vi "power data.vi"() -> ()   [LabVIEW 2014]
uses:
  <vilib>/Rock Robotics/Network Tables/NT Read Boolean Array.vi
  <vilib>/Rock Robotics/Network Tables/NT Write Boolean Array.vi
  <vilib>/Rock Robotics/Network Tables/NT Write Numeric Array.vi
  <vilib>/Rock Robotics/WPI/Power/WPI_Power Get 6Volt Rail Voltage and Current.vi
  <vilib>/Rock Robotics/WPI/Power/WPI_Power Get 5Volt Rail Voltage and Current.vi
  <vilib>/Rock Robotics/WPI/Power/WPI_Power Get 3Volt Rail Voltage and Current.vi
  typedefs/dashboard/power data.ctl
  <vilib>/Rock Robotics/Network Tables/NT Write String.vi
panel:
  out "OutputsEnabled?":bool
  out "Power (W)":dbl
  out "Energy (J)":dbl
  out "voltage (V)":dbl
  out "Hardware Fault":bool
  out "Temperature Fault":bool
  out "Battery Voltage Fault":bool
  out "Current Faults":bool[](array[boolean])
  out "all currents (A)":dbl[](array[numeric])
  out "Solenoid Voltage":dbl
  out "Input Voltage":dbl
  out "All Solenoid Faults":bool[](array[boolean])
  out "Compressor Fault":bool
  out "current (A)":dbl
  out "3.3 volt rail current (A)":dbl
  out "3.3 volt rail voltage (V)":dbl
  out "5 volt rail current (A)":dbl
  out "5 volt rail voltage (V)":dbl
  out "6 volt rail current (A)":dbl
  out "6 volt rail voltage (V)":dbl
  out "6 V User Rail Short":bool
  out "5 V User Rail Short":bool
  out "3.3V User Rail Short":bool
  out "Input Voltage Brown Out":bool
  out "roboRIO input current (A)":dbl
  out "roboRIO input voltage (V)":dbl
  # "roboRIO"
  # "General Shorts/Power"
  # "PDP"
  # "Power Rails"
  # "PCM"
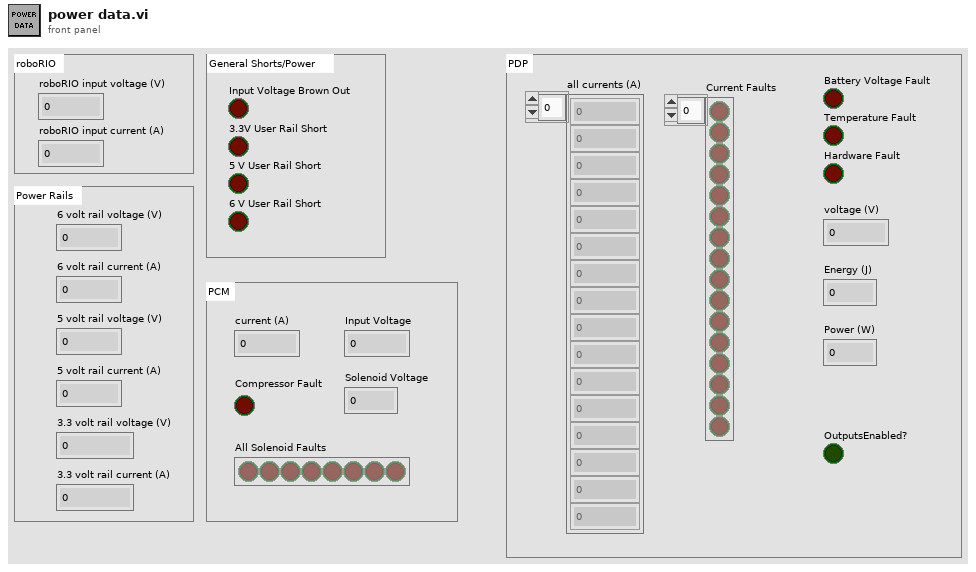
[diagram p1: front panel]
types:
  T1 = cluster{"all currents (A)":dbl[], "Current Faults":bool[], "Battery Voltage Fault":bool, "Temperature Fault":bool, "Hardware Fault":bool, "voltage (V)":dbl, "PDP Energy":cluster{"Energy (J)":dbl, "Power (W)":dbl}}
  T2 = cluster{"current (A)":dbl, "Compressor Fault":bool}
  T3 = cluster{"Input Voltage":dbl, "Solenoid Voltage":dbl}
  T4 = cluster{"Compressor":cluster{"current (A)":dbl, "Compressor Fault":bool}, "All Solenoid Faults":bool[], "PCM Voltage":cluster{"Input Voltage":dbl, "Solenoid Voltage":dbl}}
  T5 = cluster{"6 volt rail":cluster{"6 volt rail voltage (V)":dbl, "6 volt rail current (A)":dbl}, "5 volt rail":cluster{"5 volt rail voltage (V)":dbl, "5 volt rail current (A)":dbl}, "3.3 volt rail":cluster{"3.3 volt rail voltage (V)":dbl, "3.3 volt rail current (A)":dbl}}
  T6 = cluster{"3.3 volt rail voltage (V)":dbl, "3.3 volt rail current (A)":dbl}
  T7 = cluster{"5 volt rail voltage (V)":dbl, "5 volt rail current (A)":dbl}
  T8 = cluster{"6 volt rail voltage (V)":dbl, "6 volt rail current (A)":dbl}
  T9 = cluster{"Input Voltage Brown Out":bool, "3.3V User Rail Short":bool, "5 V User Rail Short":bool, "6 V User Rail Short":bool}
  T10 = cluster{"roboRIO input voltage (V)":dbl, "roboRIO input current (A)":dbl}
  T11 = cluster{"roboRIO V&I":cluster{"roboRIO input voltage (V)":dbl, "roboRIO input current (A)":dbl}, "roboRIO Faults":cluster{"Input Voltage Brown Out":bool, "3.3V User Rail Short":bool, "5 V User Rail Short":bool, "6 V User Rail Short":bool}}
  T12 = typedef "power data.ctl" = cluster{"roboRIO":cluster{"roboRIO V&I":cluster{"roboRIO input voltage (V)":dbl, "roboRIO input current (A)":dbl}, "roboRIO Faults":cluster{"Input Voltage Brown Out":bool, "3.3V User Rail Short":bool, "5 V User Rail Short":bool, "6 V User Rail Short":bool}}, "Rail Voltages":cluster{"6 volt rail":cluster{"6 volt rail voltage (V)":dbl, "6 volt rail current (A)":dbl}, "5 volt rail":cluster{"5 volt rail voltage (V)":dbl, "5 volt rail current (A)":dbl}, "3.3 volt rail":cluster{"3.3 volt rail voltage (V)":dbl, "3.3 volt rail current (A)":dbl}}, "PCM":cluster{"Compressor":cluster{"current (A)":dbl, "Compressor Fault":bool}, "All Solenoid Faults":bool[], "PCM Voltage":cluster{"Input Voltage":dbl, "Solenoid Voltage":dbl}}, "PDP":cluster{"all currents (A)":dbl[], "Current Faults":bool[], "Battery Voltage Fault":bool, "Temperature Fault":bool, "Hardware Fault":bool, "voltage (V)":dbl, "PDP Energy":cluster{"Energy (J)":dbl, "Power (W)":dbl}}, "OutputsEnabled?":bool}
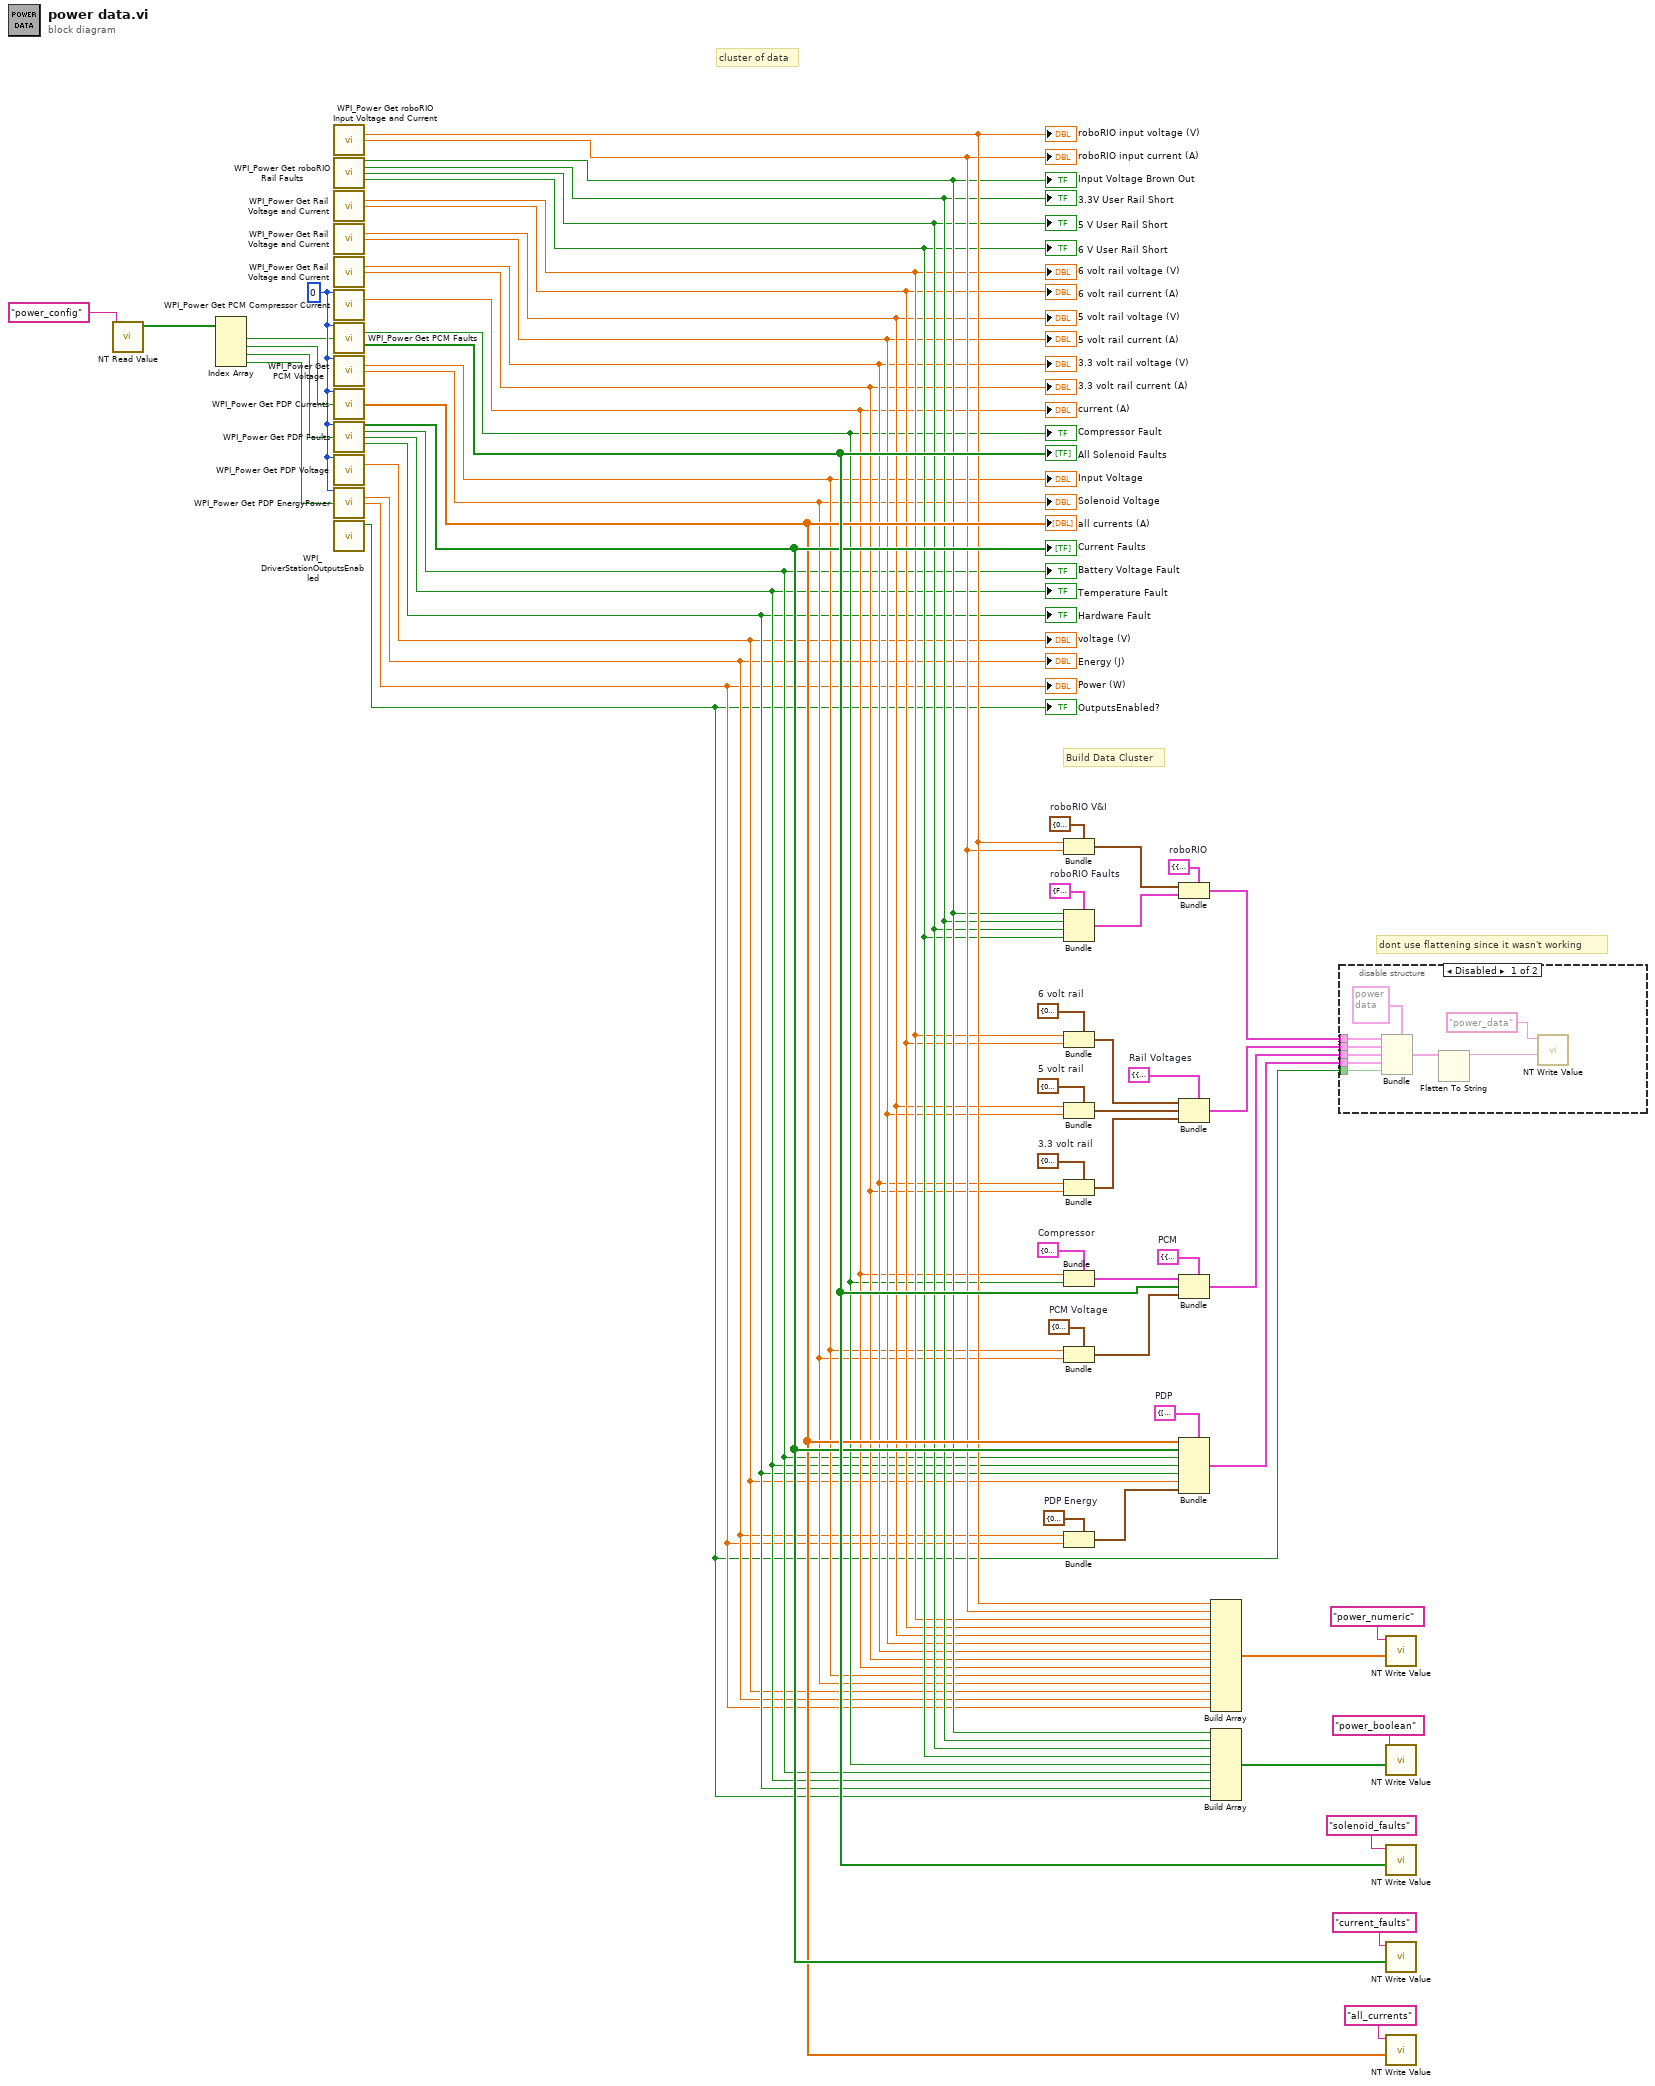
[diagram p0: block diagram]
diagram:
  w45 = cluster{"Energy (J)":dbl, "Power (W)":dbl} {"Energy (J)"=0.0, "Power (W)"=0.0}  # PDP Energy
  w46 = T1 {"all currents (A)"=[], "Current Faults"=[], "Battery Voltage Fault"=FALSE, "Temperature Fault"=FALSE, "Hardware Fault"=FALSE, "voltage (V)"=0.0, "PDP Energy"={"Energy (J)"=0.0, "Power (W)"=0.0}}  # PDP
  w50 = T2 {"current (A)"=0.0, "Compressor Fault"=FALSE}  # Compressor
  w49 = T3 {"Input Voltage"=0.0, "Solenoid Voltage"=0.0}  # PCM Voltage
  w51 = T4 {"Compressor"={"current (A)"=0.0, "Compressor Fault"=FALSE}, "All Solenoid Faults"=[], "PCM Voltage"={"Input Voltage"=0.0, "Solenoid Voltage"=0.0}}  # PCM
  w55 = T5 {"6 volt rail"={"6 volt rail voltage (V)"=0.0, "6 volt rail current (A)"=0.0}, "5 volt rail"={"5 volt rail voltage (V)"=0.0, "5 volt rail current (A)"=0.0}, "3.3 volt rail"={"3.3 volt rail voltage (V)"=0.0, "3.3 volt rail current (A)"=0.0}}  # Rail Voltages
  w58 = T6 {"3.3 volt rail voltage (V)"=0.0, "3.3 volt rail current (A)"=0.0}  # 3.3 volt rail
  w57 = T7 {"5 volt rail voltage (V)"=0.0, "5 volt rail current (A)"=0.0}  # 5 volt rail
  w56 = T8 {"6 volt rail voltage (V)"=0.0, "6 volt rail current (A)"=0.0}  # 6 volt rail
  w62 = T9 {"Input Voltage Brown Out"=FALSE, "3.3V User Rail Short"=FALSE, "5 V User Rail Short"=FALSE, "6 V User Rail Short"=FALSE}  # roboRIO Faults
  w63 = T10 {"roboRIO input voltage (V)"=0.0, "roboRIO input current (A)"=0.0}  # roboRIO V&I
  w61 = T11 {"roboRIO V&I"={"roboRIO input voltage (V)"=0.0, "roboRIO input current (A)"=0.0}, "roboRIO Faults"={"Input Voltage Brown Out"=FALSE, "3.3V User Rail Short"=FALSE, "5 V User Rail Short"=FALSE, "6 V User Rail Short"=FALSE}}  # roboRIO
  w64 = u8 0 ("Pneumatics Control Module (0)")
  # "dont use flattening since it wasn't working"
  # "Build Data Cluster"
  # "cluster of data"
  n1 = call-poly <vilib>:"NT Read Value.vi"("Name"="power_config") -> ("Boolean Array"=w5:bool[])  [unwired: 9 in, 1 out]
  n2 = Index Array(array=w5) -> (element #1=w4:bool, element #2=w3:bool, element #3=w2:bool, element #4=w1:bool)  [unwired: 4 in]
  n3 = call <vilib>:"WPI_Power Get roboRIO Input Voltage and Current.vi"() -> ("roboRIO input voltage (V)"=w29:dbl, "roboRIO input current (A)"=w28:dbl)  [unwired: 13 in, 1 out]
  "roboRIO input voltage (V)" <- w29
  "roboRIO input current (A)" <- w28
  n4 = call <vilib>:"WPI_Power Get roboRIO Rail Faults.vi"() -> ("Input Voltage Brown Out"=w27:bool, "3.3V User Rail Short"=w26:bool, "5 V User Rail Short"=w25:bool, "6 V User Rail Short"=w24:bool)  [unwired: 11 in, 1 out]
  "Input Voltage Brown Out" <- w27
  "3.3V User Rail Short" <- w26
  "5 V User Rail Short" <- w25
  "6 V User Rail Short" <- w24
  n5 = call-poly <vilib>:"WPI_Power Get Rail Voltage and Current.vi"() -> ("6 volt rail voltage (V)"=w23:dbl, "6 volt rail current (A)"=w22:dbl)  [unwired: 13 in, 1 out]
  "6 volt rail voltage (V)" <- w23
  "6 volt rail current (A)" <- w22
  n6 = call-poly <vilib>:"WPI_Power Get Rail Voltage and Current.vi"() -> ("5 volt rail voltage (V)"=w21:dbl, "5 volt rail current (A)"=w20:dbl)  [unwired: 13 in, 1 out]
  "5 volt rail voltage (V)" <- w21
  "5 volt rail current (A)" <- w20
  n7 = call-poly <vilib>:"WPI_Power Get Rail Voltage and Current.vi"() -> ("3.3 volt rail voltage (V)"=w19:dbl, "3.3 volt rail current (A)"=w18:dbl)  [unwired: 13 in, 1 out]
  "3.3 volt rail voltage (V)" <- w19
  "3.3 volt rail current (A)" <- w18
  n8 = call <vilib>:"WPI_Power Get PCM Compressor Current.vi"("Pneumatics Control Module (0)"=w64) -> ("current (A)"=w17:dbl)  [unwired: 13 in, 1 out]
  "current (A)" <- w17
  n9 = call <vilib>:"WPI_Power Get PCM Faults.vi"("Pneumatics Control Module (0)"=w64, "Clear Sticky Faults"=w4) -> ("Compressor Fault"=w16:bool, "All Solenoid Faults"=w34:bool[])  [unwired: 10 in, 2 out]
  "Compressor Fault" <- w16
  "All Solenoid Faults" <- w34
  n10 = call <vilib>:"WPI_Power Get PCM Voltage.vi"("Pneumatics Control Module (0)"=w64) -> ("Input Voltage"=w15:dbl, "Solenoid Voltage"=w14:dbl)  [unwired: 12 in, 1 out]
  "Input Voltage" <- w15
  "Solenoid Voltage" <- w14
  n11 = call <vilib>:"WPI_Power Get PDP Currents.vi"("Power Distribution Panel (0)"=w64, "Tare Currents?"=w3) -> ("all currents (A)"=w32:dbl[])  [unwired: 11 in, 2 out]
  "all currents (A)" <- w32
  n12 = call <vilib>:"WPI_Power Get PDP Faults.vi"("Power Distribution Panel (0)"=w64, "Clear Sticky Faults"=w2) -> ("Current Faults"=w33:bool[], "Battery Voltage Fault"=w13:bool, "Temperature Fault"=w12:bool, "Hardware Fault"=w11:bool)  [unwired: 9 in, 1 out]
  "Current Faults" <- w33
  "Battery Voltage Fault" <- w13
  "Temperature Fault" <- w12
  "Hardware Fault" <- w11
  n13 = call <vilib>:"WPI_Power Get PDP Voltage.vi"("Power Distribution Panel (0)"=w64) -> ("voltage (V)"=w10:dbl)  [unwired: 13 in, 1 out]
  "voltage (V)" <- w10
  n14 = call <vilib>:"WPI_Power Get PDP EnergyPower.vi"("Power Distribution Panel (0)"=w64, "Reset Energy?"=w1) -> ("Energy (J)"=w9:dbl, "Power (W)"=w8:dbl)  [unwired: 11 in, 1 out]
  "Energy (J)" <- w9
  "Power (W)" <- w8
  n15 = call <vilib>:"WPI_DriverStationOutputsEnabled.vi"() -> ("OutputsEnabled?"=w7:bool)  [unwired: 10 in, 1 out]
  "OutputsEnabled?" <- w7
  n16 = Bundle(cluster=w63, "roboRIO input voltage (V)"=w29, "roboRIO input current (A)"=w28) -> (w60:T10)
  n17 = Bundle(cluster=w62, "Input Voltage Brown Out"=w27, "3.3V User Rail Short"=w26, "5 V User Rail Short"=w25, "6 V User Rail Short"=w24) -> (w59:T9)
  n18 = Bundle(cluster=w56, "6 volt rail voltage (V)"=w23, "6 volt rail current (A)"=w22) -> (w54:T8)
  n19 = Bundle(cluster=w57, "5 volt rail voltage (V)"=w21, "5 volt rail current (A)"=w20) -> (w53:T7)
  n20 = Bundle(cluster=w58, "3.3 volt rail voltage (V)"=w19, "3.3 volt rail current (A)"=w18) -> (w52:T6)
  n21 = Bundle(cluster=w50, "current (A)"=w17, "Compressor Fault"=w16) -> (w48:T2)
  n22 = Bundle(cluster=w49, "Input Voltage"=w15, "Solenoid Voltage"=w14) -> (w47:T3)
  n23 = Bundle(cluster=w45, "Energy (J)"=w9, "Power (W)"=w8) -> (w44:cluster{"Energy (J)":dbl, "Power (W)":dbl})
  n24 = Bundle(cluster=w61, "roboRIO V&I"=w60, "roboRIO Faults"=w59) -> (w43:T11)
  n25 = Bundle(cluster=w55, "6 volt rail"=w54, "5 volt rail"=w53, "3.3 volt rail"=w52) -> (w42:T5)
  n26 = Bundle(cluster=w51, "Compressor"=w48, "All Solenoid Faults"=w34, "PCM Voltage"=w47) -> (w41:T4)
  n27 = Bundle(cluster=w46, "all currents (A)"=w32, "Current Faults"=w33, "Battery Voltage Fault"=w13, "Temperature Fault"=w12, "Hardware Fault"=w11, "voltage (V)"=w10, "PDP Energy"=w44) -> (w40:T1)
  n28 = Build Array(w29, w28, w23, w22, w21, w20, w19, w18, w17, w15, w14, w10, w9, w8) -> (w30:dbl[])
  n29 = Build Array(w27, w26, w25, w24, w16, w13, w12, w11, w7) -> (w31:bool[])
  n30 = disable-structure shown="Disabled" {
    disable-tunnel: w43 -> [w72 _]
    disable-tunnel: w42 -> [w71 _]
    disable-tunnel: w41 -> [w70 _]
    disable-tunnel: w40 -> [w69 _]
    disable-tunnel: w7 -> [w68 _]
    frame Disabled {
      n31 = Bundle(cluster=T12 {"roboRIO"={"roboRIO V&I"={"roboRIO input voltage (V)"=0.0, "roboRIO input current (A)"=0.0}, "roboRIO Faults"={"Input Voltage Brown Out"=FALSE, "3.3V User Rail Short"=FALSE, "5 V User Rail Short"=FALSE, "6 V User Rail Short"=FALSE}}, "Rail Voltages"={"6 volt rail"={"6 volt rail voltage (V)"=0.0, "6 volt rail current (A)"=0.0}, "5 volt rail"={"5 volt rail voltage (V)"=0.0, "5 volt rail current (A)"=0.0}, "3.3 volt rail"={"3.3 volt rail voltage (V)"=0.0, "3.3 volt rail current (A)"=0.0}}, "PCM"={"Compressor"={"current (A)"=0.0, "Compressor Fault"=FALSE}, "All Solenoid Faults"=[], "PCM Voltage"={"Input Voltage"=0.0, "Solenoid Voltage"=0.0}}, "PDP"={"all currents (A)"=[], "Current Faults"=[], "Battery Voltage Fault"=FALSE, "Temperature Fault"=FALSE, "Hardware Fault"=FALSE, "voltage (V)"=0.0, "PDP Energy"={"Energy (J)"=0.0, "Power (W)"=0.0}}, "OutputsEnabled?"=FALSE} ("Power Data"), "roboRIO"=w72, "Rail Voltages"=w71, "PCM"=w70, "PDP"=w69, "OutputsEnabled?"=w68) -> (w67:T12)
      n32 = Flatten To String(anything=w67) -> (data string=w65:string)  [unwired: 3 in, 2 out]
      n33 = call-poly <vilib>:"NT Write Value.vi"("String"=w65, "Name"="power_data") -> ()  [unwired: 9 in, 1 out]
    }
    frame Enabled {
    }
  }
  n34 = call-poly <vilib>:"NT Write Value.vi"("Numeric Array"=w30, "Name"="power_numeric") -> ()  [unwired: 9 in, 1 out]
  n35 = call-poly <vilib>:"NT Write Value.vi"("Boolean Array"=w31, "Name"="power_boolean") -> ()  [unwired: 9 in, 1 out]
  n36 = call-poly <vilib>:"NT Write Value.vi"("Boolean Array"=w34, "Name"="solenoid_faults") -> ()  [unwired: 9 in, 1 out]
  n37 = call-poly <vilib>:"NT Write Value.vi"("Boolean Array"=w33, "Name"="current_faults") -> ()  [unwired: 9 in, 1 out]
  n38 = call-poly <vilib>:"NT Write Value.vi"("Numeric Array"=w32, "Name"="all_currents") -> ()  [unwired: 9 in, 1 out]
